vi "get_or_set_position_feedback.vi"(7 "action":T1, 8 "error in (no error)":errorcluster, 10 "position feedback data in":T2, 11 "ScanHeadDL090202 in":refnum<class "ScanHeadDL090202.lvclass">) -> (0 "error out":errorcluster, 2 "position feedback data out":T2, 3 "ScanHeadDL090202 out":refnum<class "ScanHeadDL090202.lvclass">)   [LabVIEW 2010, in "ScanHeadDL090202.lvclass"]
uses:
  ScanHeadDL090202.lvclass
  common/arrays/pixel_raw_data_array.ctl
  common/enumerations/functional_global_action_enum.ctl
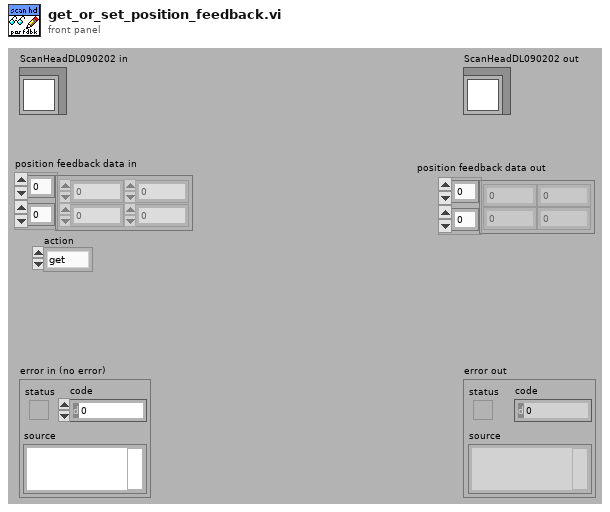
[diagram p1: front panel]
types:
  T1 = typedef "functional_global_action_enum.ctl" = enum16{"get", "set", "reset"}
  T2 = typedef "pixel_raw_data_array.ctl" = dbl[][]
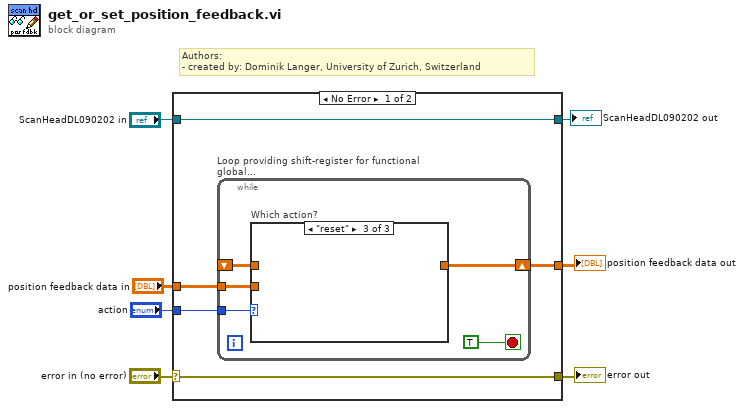
[diagram p0: block diagram]
diagram:
  # "Authors: \n- created by: Dominik Langer, University of Zurich, Switzerland"
  n1 = case shown="No Error" "error in (no error)" {
    selector: "error in (no error)" -> [w10 w21]
    tunnel: [w10 w21] -> w6
    tunnel: [w12 w20] -> w4
    tunnel: "ScanHeadDL090202 in" -> [w12 w20]
    tunnel: "action" -> [w11 _]
    tunnel: "position feedback data in" -> [w9 _]
    tunnel: [w8 _] -> w1
    frame No Error {
      n2 = while "Loop providing shift-register for functional global..." {
        shift-right: [w14] -> w8
        shift-left: _ -> [w13]
        tunnel: w11 -> [w16]
        tunnel: w9 -> [w15]
        stop <- TRUE stop-if-true
        n3 = case "Which action?" shown="\"reset\"" w16 {
          tunnel: w15 -> [_ w19 _]
          tunnel: [w18 w19 _] -> w14
          tunnel: w13 -> [w18 _ _]
          frame "get", Default {
          }
          frame "set" {
          }
          frame "reset" {
          }
        }
      }
    }
    frame Error {
    }
  }
  "error out" <- w6
  "ScanHeadDL090202 out" <- w4
  "position feedback data out" <- w1
